vi "Stop.vi"(8 "error in (no error)":errorcluster, 11 "NI DAQmx Base in":refnum<class "NI DAQmx Base.lvclass">) -> (0 "error out":errorcluster, 3 "NI DAQmx Base out":refnum<class "NI DAQmx Base.lvclass">)   [LabVIEW 2020, in "NI DAQmx.lvlib" / "NI DAQmx Base.lvclass"]
uses:
  NI DAQmx Base.lvclass
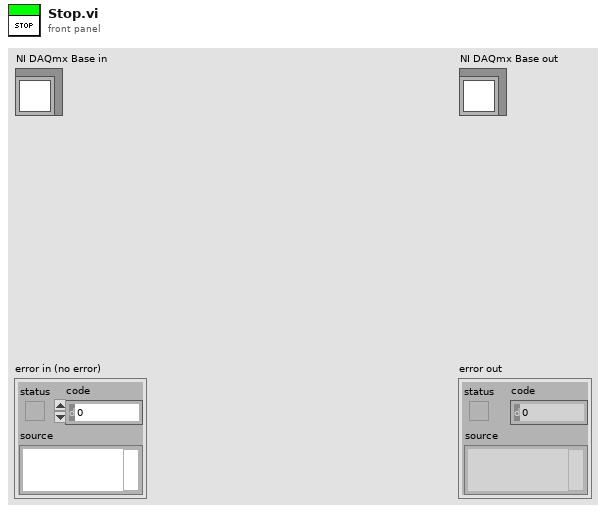
[diagram p1: front panel]
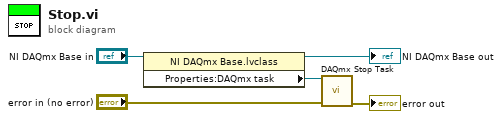
[diagram p0: block diagram]
diagram:
  n1 = property class="NI DAQmx Base.lvclass"(reference="NI DAQmx Base in") -> (reference out=→"NI DAQmx Base out":refnum<class "NI DAQmx Base.lvclass">, "Properties:DAQmx task"=w5:refnum<k21>)  [unwired: 1 in, 1 out]
  n2 = call <vilib>:"DAQmx Stop Task.vi"("task/channels in"=w5, "error in"="error in (no error)") -> ("error out"=→"error out":errorcluster)  [unwired: 12 in, 1 out]
